vi "UE9 LJTDAC Example.vi"(9 "DACB":dbl step=0.1 format="%.4f", 10 "DACA":dbl step=0.1 format="%.4f", 11 "SCL Pin #":i32) -> (0 "error out":errorcluster)   [LabVIEW 2021]
panel:
  in  "FirstFound":bool=TRUE
  in  "ConnectionType":u16(ring) items=["LJ_ctUSB", "LJ_ctETHERNET"]
  in  "Address":string="192.168.1.209"
  out "Error Message":string
  # "Specify an IP address for Ethernet, or Local ID\nfor USB.  If FirstFound is selected, Local ID is\nignored for USB."
  # "Updates both channels on an LJTick-DAC."
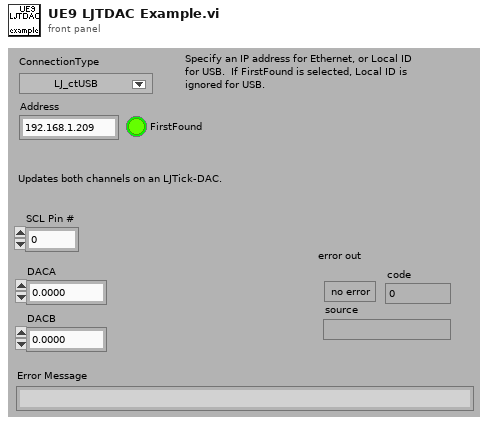
[diagram p1: front panel]
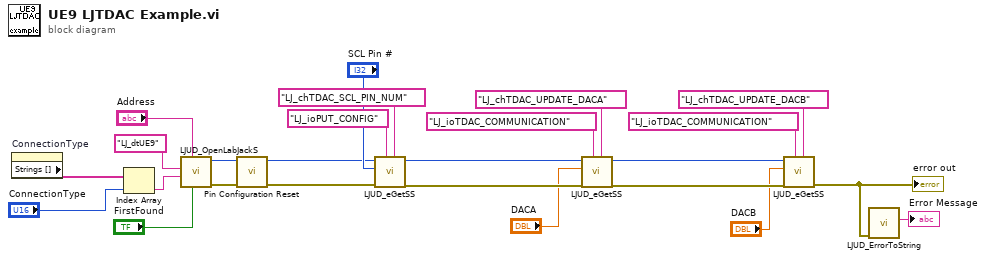
[diagram p0: block diagram]
diagram:
  n1 = property on="ConnectionType" class="Ring (strict)"() -> ("Strings []"=w3:string[])  [unwired: 2 in, 2 out]
  n2 = Index Array(array=w3, index="ConnectionType") -> (element=w2:string)
  n3 = call "LJUD_OpenLabJackS.vi"("FirstFound"="FirstFound", "Address"="Address", "ConnectionType"=w2, "DeviceType"="LJ_dtUE9") -> ("error out"=w22:errorcluster, "Handle"=w23:i32)  [unwired: 5 in, 1 out]
  n4 = call "Pin Configuration Reset.vi"("error in"=w22, "Handle In"=w23) -> ("error out"=w17:errorcluster, "Handle Out"=w18:i32)  [unwired: 8 in]
  n5 = call "LJUD_eGetSS.vi"("Channel"="LJ_chTDAC_SCL_PIN_NUM", "IOType"="LJ_ioPUT_CONFIG", "error in"=w17, "Value Write"="SCL Pin #", "Handle In"=w18) -> ("error out"=w13:errorcluster, "Handle Out"=w14:i32)  [unwired: 4 in, 1 out]
  n6 = call "LJUD_eGetSS.vi"("Channel"="LJ_chTDAC_UPDATE_DACA", "IOType"="LJ_ioTDAC_COMMUNICATION", "error in"=w13, "Value Write"="DACA", "Handle In"=w14) -> ("error out"=w8:errorcluster, "Handle Out"=w9:i32)  [unwired: 4 in, 1 out]
  n7 = call "LJUD_eGetSS.vi"("Channel"="LJ_chTDAC_UPDATE_DACB", "IOType"="LJ_ioTDAC_COMMUNICATION", "error in"=w8, "Value Write"="DACB", "Handle In"=w9) -> ("error out"=w7:errorcluster)  [unwired: 4 in, 2 out]
  "error out" <- w7
  n8 = call "LJUD_ErrorToString.vi"("error in"=w7) -> ("String"=→"Error Message":string)  [unwired: 10 in]
